vi "F Dwf Digital Spi Order Set.vi"(8 "error in (no error)":errorcluster, 10 "fMSBFirst":i32, 11 "hdwf":i32) -> (0 "error out":errorcluster, 3 "function return":i32)   [LabVIEW 2021, in "Olasdwf.lvlib"]
doc: "DWFAPI int FDwfDigitalSpiDataSet(HDWF hdwf, int idxDQ, int idxChannel); DWFAPI int FDwfDigitalSpiModeSet(HDWF hdwf, int iMode); DWFAPI int FDwfDigitalSpiOrderSet(HDWF hdwf, int fMSBFirst);"
uses:
  Olasdwf.lvlib
  Windows/System32/dwf.dll
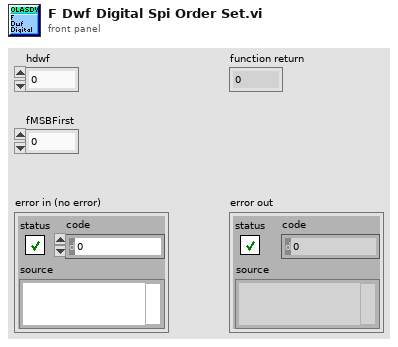
[diagram p1: front panel]
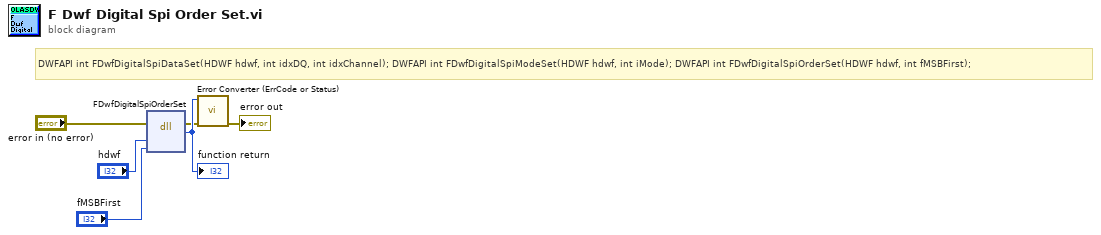
[diagram p0: block diagram]
diagram:
  # "DWFAPI int FDwfDigitalSpiDataSet(HDWF hdwf, int idxDQ, int idxChannel); DWFAPI int FDwfDigitalSpiModeSet(HDWF hdwf, int iMode); DWFAPI int FDwfDigitalSpiOrderSet(HDWF hdwf, int fMSBFirst);"
  n1 = dll-call lib="/Windows/System32/dwf.*" fn="FDwfDigitalSpiOrderSet"(error in="error in (no error)", "hdwf"="hdwf", "fMSBFirst"="fMSBFirst") -> (error out=w2:errorcluster, w6:i32)  [unwired: 4 in, 1 out]
  "function return" <- w6
  n2 = call "Error Converter (ErrCode or Status).vi"("error in (no error)"=w2, "error code"=w6) -> ("error out"=→"error out":errorcluster)  [unwired: 9 in]
